vi "Delete Notification By Handle.vi"(8 "error in (no error)":errorcluster, 10 "Handle":i32, 11 "TwinCAT ADS in":refnum<class "TwinCAT ADS.lvclass">) -> (0 "error out":errorcluster, 3 "TwinCAT ADS out":refnum<class "TwinCAT ADS.lvclass">)   [LabVIEW 2018, in "TwinCAT ADS.lvclass"]
uses:
  TwinCAT ADS.lvclass
  TwinCAT ADS.lvclass/TwinCAT ADS.ctl
  TwinCAT.Ads
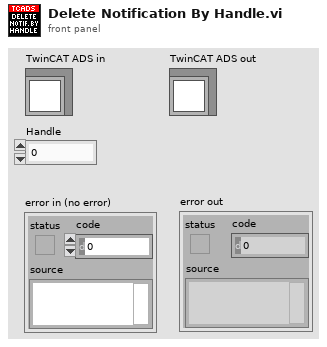
[diagram p1: front panel]
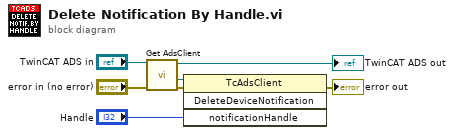
[diagram p0: block diagram]
diagram:
  n1 = call "Get AdsClient.vi"("error in (no error)"="error in (no error)", "TwinCAT ADS in"="TwinCAT ADS in") -> ("error out"=w5:errorcluster, ".NET TcAdsClient"=w4:refnum<k24>, "TwinCAT ADS out"=→"TwinCAT ADS out":refnum<class "TwinCAT ADS.lvclass">)  [unwired: 7 in]
  n2 = invoke class="TcAdsClient" method="DeleteDeviceNotification"(reference=w4, error in=w5, "notificationHandle"="Handle") -> (error out=→"error out":errorcluster)  [unwired: 1 in, 3 out]
